vi "PathPlanner_Constraints_FromJSON.vi"(11 "JSON Object":string) -> (3 "ConstraintsZone":T1)   [LabVIEW 2019, in "PathPlanner24.lvlib"]
doc: "/**\n * Create a path constraints object from json\n *\n * @param constraintsJson {@link org.json.simple.JSONObject} representing a path constraints\n * object\n * @return The path constraints defined by the given json\n */"
uses:
  PathPlanner24.lvlib
  TypeDef/PathPlannerConstraints.ctl
  TypeDef/PathPlannerConstraintsZone.ctl
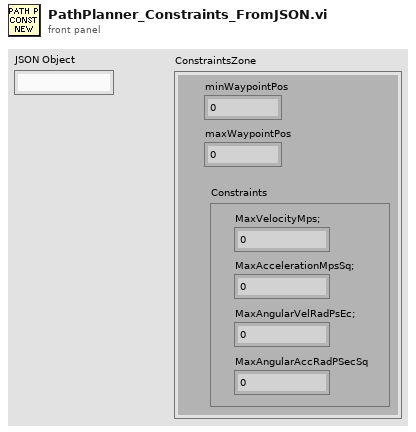
[diagram p1: front panel]
types:
  T1 = typedef "PathPlanner24.lvlib/PathPlannerConstraintsZone.ctl" = cluster{"minWaypointPos":dbl, "maxWaypointPos":dbl, "Constraints":T2}
  T2 = typedef "PathPlanner24.lvlib/PathPlannerConstraints.ctl" = cluster{"MaxVelocityMps;":dbl, "MaxAccelerationMpsSq;":dbl, "MaxAngularVelRadPsEc;":dbl, "MaxAngularAccRadPSecSq":dbl}
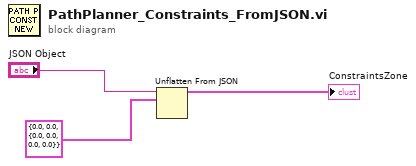
[diagram p0: block diagram]
diagram:
  n1 = Unflatten From JSON(JSON string="JSON Object", type and defaults=T1 {"minWaypointPos"=0.0, "maxWaypointPos"=0.0, "Constraints"={"MaxVelocityMps;"=0.0, "MaxAccelerationMpsSq;"=0.0, "MaxAngularVelRadPsEc;"=0.0, "MaxAngularAccRadPSecSq"=0.0}} ("ConstraintsZone")) -> (value=→"ConstraintsZone":T1)  [unwired: 5 in, 1 out]
